vi "ImageAvailalbeMain.vi"() -> ()   [LabVIEW 2017]
panel:
  in  "stop":bool
  in  "ICImagingControl":refnum<k7>(container)
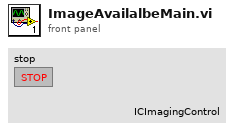
[diagram p1: front panel]
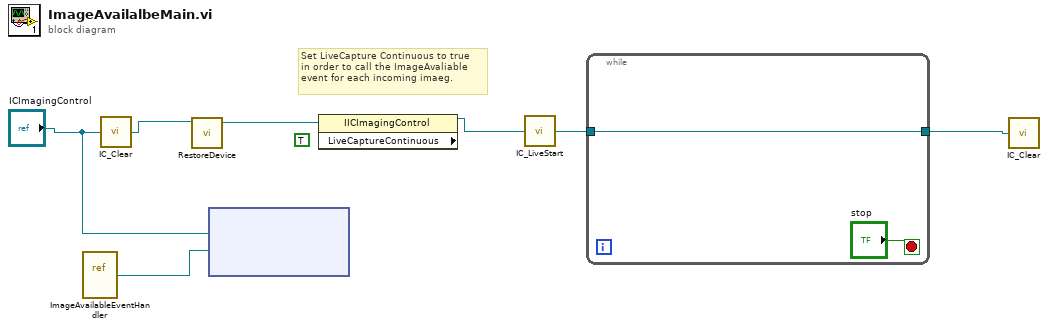
[diagram p0: block diagram]
diagram:
  (unwired) TRUE ("LiveCaptureContinuous")
  # "Set LiveCapture Continuous to true\nin order to call the ImageAvaliable\nevent for each incoming imaeg."
  n1 = vi-ref "ImageAvailableEventHandler.vi"() -> ("vi reference"=w1:refnum<vi>)
  n2 = call <userlib>:"IC_Clear.vi"("ICImagingControl 2"="ICImagingControl") -> ("ICImagingControl"=w7:refnum<k7>)
  n3 = call <userlib>:"RestoreDevice.vi"("ICImagingControl"=w7) -> ("ICImagingControl 2"=w6:refnum<k7>)  [unwired: 3 in, 2 out]
  n4 = node("ICImagingControl", w1) -> ()  [unwired: 3 in, 2 out]
  n5 = property class="IICImagingControl" props=["LiveCaptureContinuous"](reference=w6) -> (reference out=w5:refnum<k7>)  [unwired: 1 in, 2 out]
  n6 = call <userlib>:"IC_LiveStart.vi"("ICImagingControl 3"=w5) -> ("ICImagingControl 2"=w4:refnum<k7>)
  n7 = while {
    tunnel: w4 -> [w8]
    tunnel: [w8] -> w3
    stop <- "stop" stop-if-true
  }
  n8 = call <userlib>:"IC_Clear.vi"("ICImagingControl 2"=w3) -> ()  [unwired: 1 out]
